vi "数据查询_仪器数据.vi"() -> ()   [LabVIEW 2016]
uses:
  <vilib>/Utility/miscctls.llb/LVPointTypeDef.ctl
  <vilib>/Utility/miscctls.llb/LVRowAndColumnUnsignedTypeDef.ctl
  <userlib>/_OpenG.lib/array/array.llb/Sort 2D Array (String)__ogtk.vi
panel:
  in  "序列号":string
  in  "关闭":bool
  in  "导出":bool
  out "分钟小时":string(combo)="实时数据"
  out "工作类型":string(combo)="全部数据"
  in  "工作模式":string(combo)="全部数据"
  in  "查询":bool
  in  "结束日期":string="2020/01/01"
  in  "起始日期":string="2010/01/01"
  in  "组合框":string(combo)
  out "数据表":string[][](table)
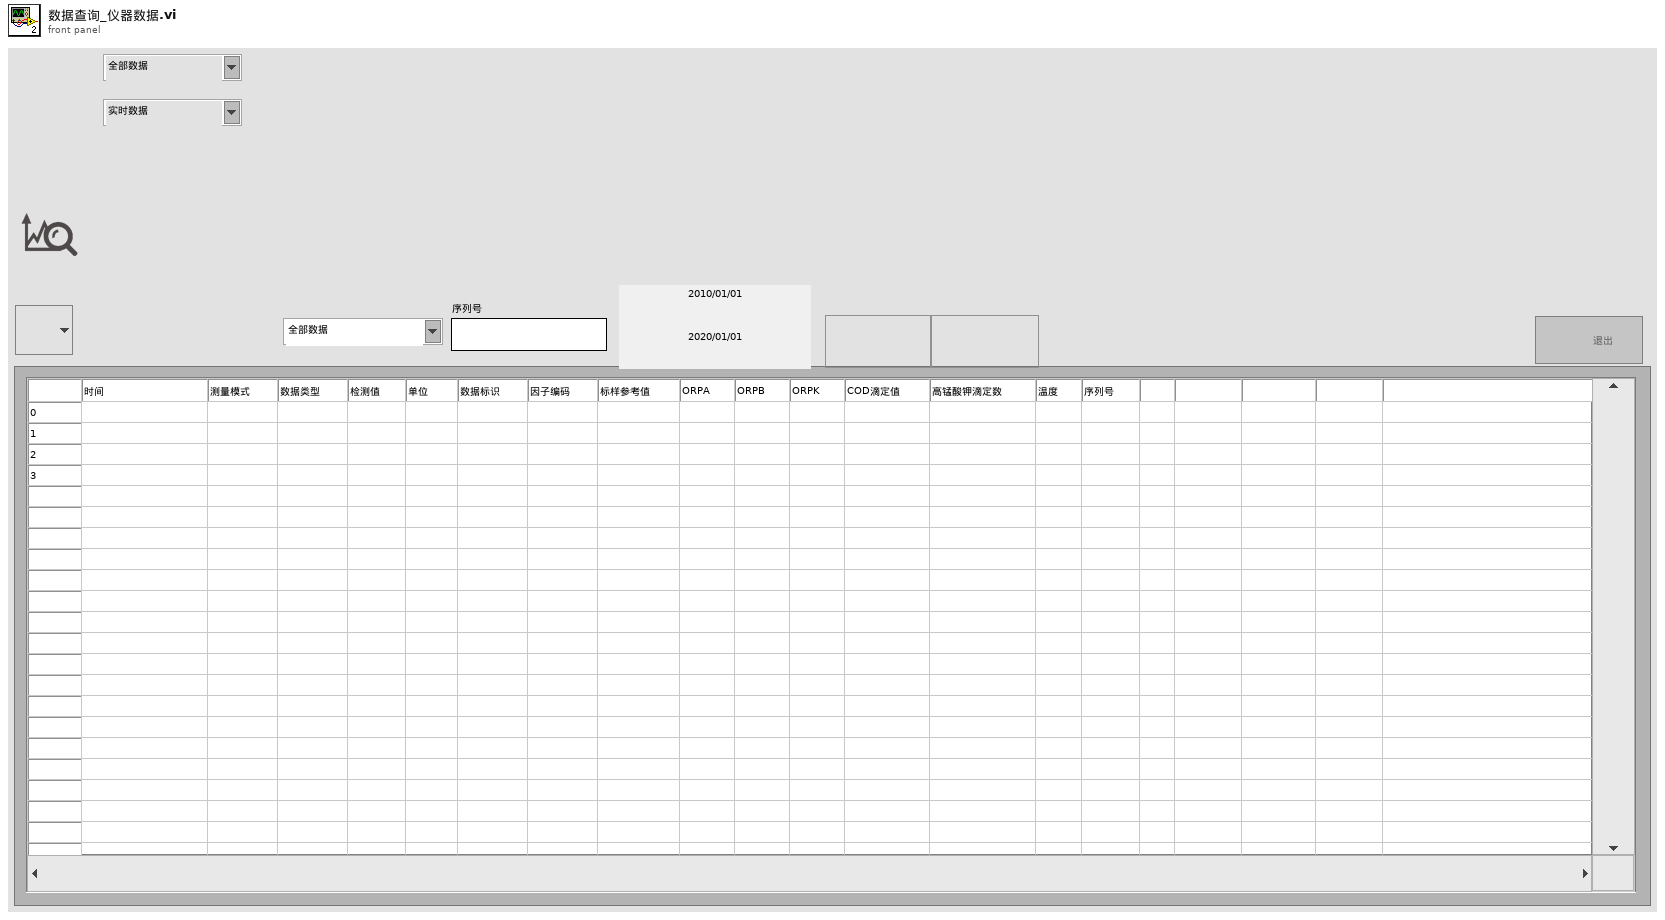
[diagram p1: front panel]
types:
  T1 = enum8{"Enabled", "Disabled", "Disabled and Grayed Out"}
  T2 = typedef "LVRowAndColumnUnsignedTypeDef.ctl" = cluster{"Row":u32, "Column":u32}
  T3 = typedef "LVPointTypeDef.ctl" = cluster{"Horizontal":i16, "Vertical":i16}
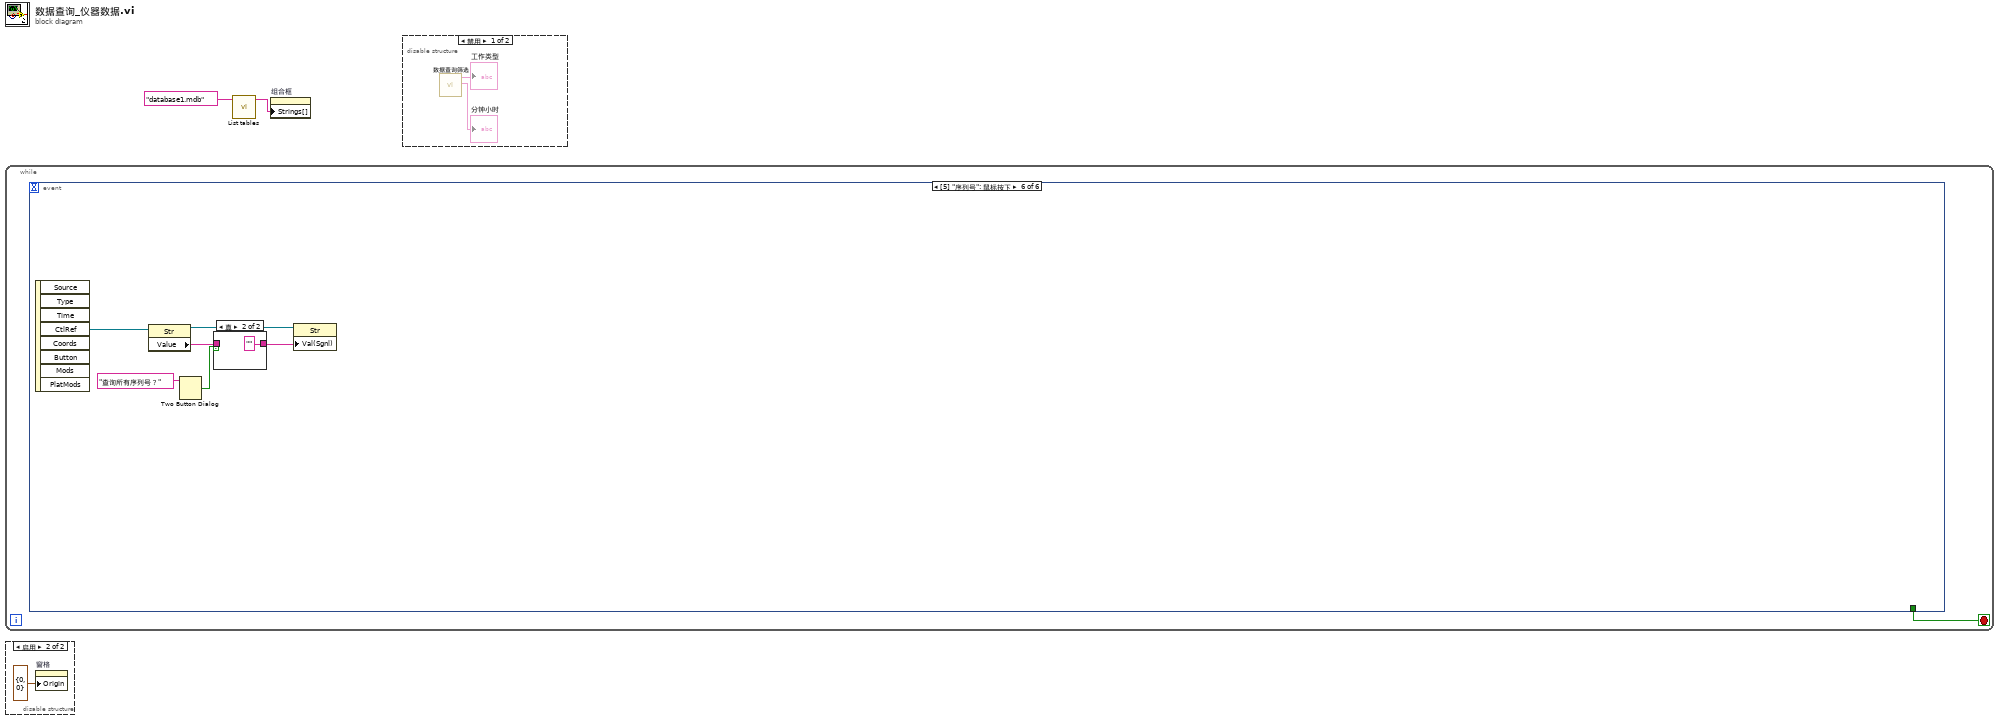
[diagram p0: block diagram]
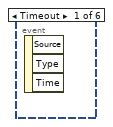
[diagram p3: hidden frame]
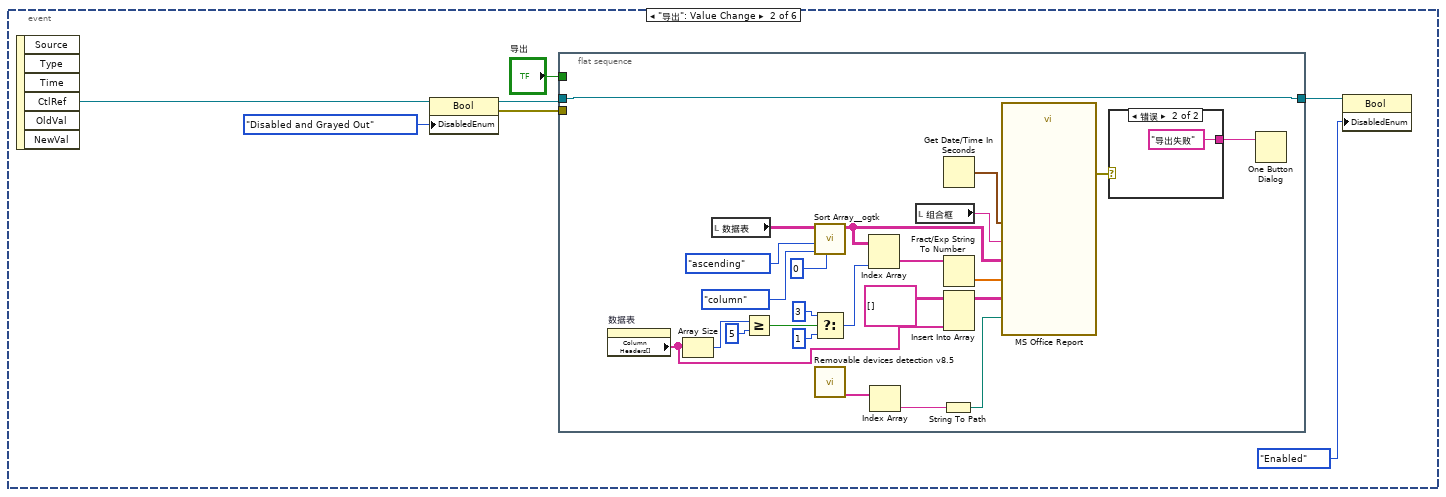
[diagram p4: hidden frame]
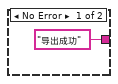
[diagram p5: hidden frame]
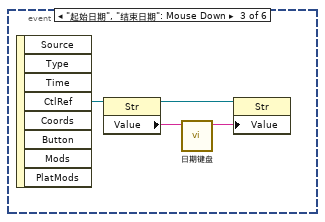
[diagram p6: hidden frame]
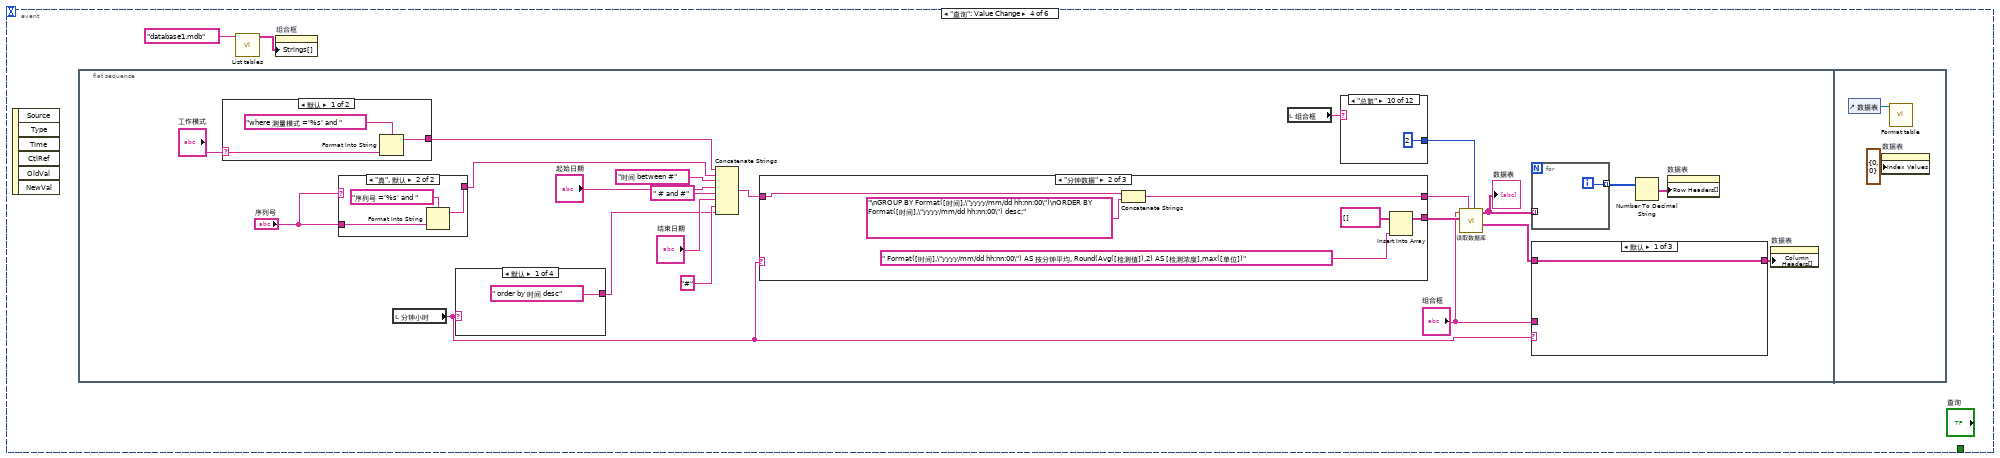
[diagram p7: hidden frame]
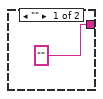
[diagram p8: hidden frame]
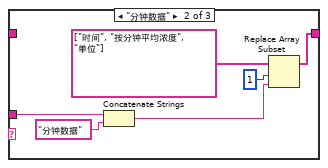
[diagram p9: hidden frame]
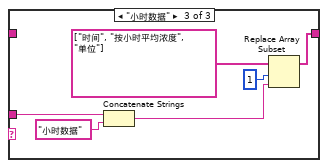
[diagram p10: hidden frame]
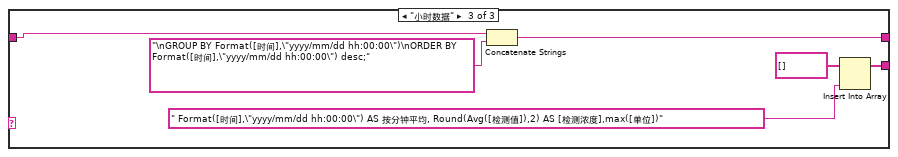
[diagram p15: hidden frame]
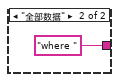
[diagram p16: hidden frame]
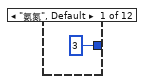
[diagram p17: hidden frame]
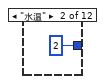
[diagram p18: hidden frame]
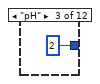
[diagram p19: hidden frame]
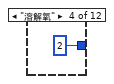
[diagram p20: hidden frame]
diagram:
  n1 = while {
    stop <- w3 stop-if-true
    n2 = event shown="[5] \"序列号\": 鼠标按下" {
      selector: _ -> [_ _ _ _ _ _]
      dyn-events: _ -> [_ _ _ _ _ _]
      timeout: _ -> [_ _ _ _ _ _]
      tunnel: [_ _ _ _ TRUE ("停止？(T)") _] -> w3
      event Timeout {
        n3 = event-data() -> ()  [unwired: 1 in, 3 out]
      }
      event "导出": Value Change {
        n4 = event-data() -> ("CtlRef"=w4:refnum<vi>)  [unwired: 1 in, 5 out]
        n5 = property class="Bool"(reference=w4, "DisabledEnum"=T1."Disabled and Grayed Out" ("禁用")) -> (reference out=w8:refnum<vi>, error out=w9:errorcluster)  [unwired: 1 in]
        n6 = flat-sequence {
          tunnel: w9 -> [_]
          tunnel: [w25] -> w7
          tunnel: w8 -> [w25]
          tunnel: "导出" -> [_]
          frame #0 {
            n7 = property on="数据表" class="Tbl (严格)"() -> ("Column Headers[]"=w12:string[])  [unwired: 2 in, 2 out]
            n8 = Array Size(array=w12) -> (size(s)=w19:i32)
            n9 = local read "数据表"() -> (w33:string[][])
            n10 = Greater Or Equal?(x=w19, y=5) -> (x >= y?=w17:bool)
            n11 = call-poly <userlib>:"Sort Array__ogtk.vi"("Column/Row to Sort By"=u32 0, "Sort By in"=enum16{"row", "column"}."column", "Order"=enum16{"ascending", "descending"}."ascending", "Array in"=w33) -> ("Sorted Array out"=w32:string[][])  [unwired: 4 in, 3 out]
            n12 = Select(t=3 ("禁用的索引 (列)"), s=w17, f=1) -> (s? t:f=w15:i32)
            n13 = call "Removable devices detection v8.5.vi"() -> ("Removable"=w22:string[])  [unwired: 4 out]
            n14 = Index Array(array=w32, index (col)=w15) -> (element=w28:string[])  [unwired: 1 in]
            n15 = Index Array(array=w22) -> (element=w21:string)  [unwired: 1 in]
            n16 = local read "组合框"() -> (w26:string)
            n17 = String To Path(string=w21) -> (path=w20:path)
            n18 = Get Date/Time In Seconds() -> (seconds since 1Jan1904=w34:timestamp)
            n19 = Fract/Exp String To Number(string=w28) -> (number=w27:dbl[])  [unwired: 3 in, 1 out]
            n20 = Insert Into Array(array=string[][] [], new element=w12) -> (w11:string[][])  [unwired: 2 in]
            n21 = call "MS Office Report"("Path to Save Report"=w20, "导出日期"=w34, "监测参数"=w26, "数据输入"=w32, "图表输入"=w27, "字段定义"=w11) -> ("error out"=w24:errorcluster)  [unwired: 20 in, 1 out]
            n22 = case shown="错误" w24 {
              tunnel: ["导出成功" ("消息") "导出失败" ("消息")] -> w23
              frame No Error {
              }
              frame Error {
              }
            }
            n23 = One Button Dialog(message=w23) -> ()  [unwired: 1 in, 1 out]
          }
        }
        n24 = property class="Bool"(reference=w7, "DisabledEnum"=T1."Enabled" ("禁用")) -> ()  [unwired: 1 in, 2 out]
      }
      event "起始日期", "结束日期": Mouse Down {
        n25 = event-data() -> ("CtlRef"=w40:refnum<vi>)  [unwired: 1 in, 7 out]
        n26 = property class="Str"(reference=w40) -> (reference out=w38:refnum<vi>, "Value"=w39:string)  [unwired: 1 in, 1 out]
        n27 = call "日期键盘.vi"("原值"=w39) -> ("x+y"=w37:string)  [unwired: 10 in]
        n28 = property class="Str"(reference=w38, "Value"=w37) -> ()  [unwired: 1 in, 2 out]
      }
      event "查询": Value Change {
        n29 = event-data() -> ()  [unwired: 1 in, 6 out]
        n30 = flat-sequence {
          frame #0 {
            n31 = case shown="默认" "工作模式" {
              selector: "工作模式" -> [w98 _]
              tunnel: [w96 "where " ("condition")] -> w44
              frame Default {
                n32 = Format Into String(format string="where 测量模式 ='%s' and " ("condition"), w98) -> (resulting string=w96:string)  [unwired: 2 in, 1 out]
              }
              frame "全部数据" {
              }
            }
            n33 = case shown="\"真\", 默认" "序列号" {
              tunnel: "序列号" -> [_ w67]
              tunnel: ["" ("condition") w66] -> w43
              frame "" {
              }
              frame "真", Default {
                n34 = Format Into String(format string="序列号 ='%s' and " ("condition"), w67) -> (resulting string=w66:string)  [unwired: 2 in, 1 out]
              }
            }
            n35 = local read "分钟小时"() -> (w51:string)
            n36 = case shown="默认" w51 {
              tunnel: [" order by 时间 desc" ("字符串") _ _ _] -> w55
              frame Default {
              }
              frame "分钟数据" {
              }
              frame "小时数据" {
              }
              frame "真" {
              }
            }
            n37 = Concatenate Strings(w44, w43, "时间 between #" ("condition"), "起始日期", " # and #" ("condition"), "结束日期", "#" ("condition"), w55) -> (w54:string)
            n38 = case shown="\"分钟数据\"" w51 {
              tunnel: [_ w88 w90] -> w52
              tunnel: w54 -> [w83 w86 w92]
              tunnel: [w83 w85 w91] -> w53
              frame Default {
              }
              frame "分钟数据" {
                n39 = Concatenate Strings(w86, "\nGROUP BY Format([时间],\"yyyy/mm/dd hh:nn:00\")\nORDER BY Format([时间],\"yyyy/mm/dd hh:nn:00\") desc;" ("字符串")) -> (w85:string)
                n40 = Insert Into Array(array=string[] [] ("显示项"), new element=" Format([时间],\"yyyy/mm/dd hh:nn:00\") AS 按分钟平均, Round(Avg([检测值]),2) AS [检测浓度],max([单位])" ("新元素/子数组")) -> (w88:string[])  [unwired: 1 in]
              }
              frame "小时数据" {
                n41 = Concatenate Strings(w92, "\nGROUP BY Format([时间],\"yyyy/mm/dd hh:00:00\")\nORDER BY Format([时间],\"yyyy/mm/dd hh:00:00\") desc;" ("字符串")) -> (w91:string)
                n42 = Insert Into Array(array=string[] [] ("显示项"), new element=" Format([时间],\"yyyy/mm/dd hh:00:00\") AS 按分钟平均, Round(Avg([检测值]),2) AS [检测浓度],max([单位])" ("新元素/子数组")) -> (w90:string[])  [unwired: 1 in]
              }
            }
            n43 = local read "组合框"() -> (w57:string)
            n44 = case shown="\"总氮\"" w57 {
              tunnel: [i16 3 ("精度(6)") i16 2 ("精度(6)") i16 2 ("精度(6)") i16 2 ("精度(6)") i16 2 ("精度(6)") i16 2 ("精度(6)") i16 2 ("精度(6)") i16 2 ("精度(6)") i16 3 ("精度(6)") i16 2 ("精度(6)") i16 2 ("精度(6)") i16 2 ("精度(6)")] -> w56
              frame "氨氮", Default {
              }
              frame "水温" {
              }
              frame "pH" {
              }
              frame "溶解氧" {
              }
              frame "电导率" {
              }
              frame "浊度" {
              }
              frame "藻密度" {
              }
              frame "叶绿素a" {
              }
              frame "总磷" {
              }
              frame "总氮" {
              }
              frame "CodCr" {
              }
              frame "CodMn" {
              }
            }
            n45 = call "读取数据库.vi"("精度(6)"=w56, "condition"=w53, "显示项"=w52, "组合框"="组合框") -> ("columns"=w50:string[], "表格"=w60:string[][])  [unwired: 4 in, 2 out]
            "数据表" <- w60
            n46 = for {
              tunnel: w60 -> [_] mode=indexing
              tunnel: [w112] -> w59 mode=indexing
              i -> [w112]
            }
            n47 = case shown="默认" w51 {
              tunnel: w50 -> [w69 _ _]
              tunnel: [w69 w73 w77] -> w49
              tunnel: "组合框" -> [_ w72 w78]
              frame Default {
              }
              frame "分钟数据" {
                n48 = Concatenate Strings(w72, "分钟数据" ("字符串")) -> (w70:string)
                n49 = Replace Array Subset(array=string[] ["时间", "按分钟平均浓度", "单位"] ("columns"), new element=w70, index=1 ("索引")) -> (w73:string[])
              }
              frame "小时数据" {
                n50 = Concatenate Strings(w78, "小时数据" ("字符串")) -> (w79:string)
                n51 = Replace Array Subset(array=string[] ["时间", "按小时平均浓度", "单位"] ("columns"), new element=w79, index=1 ("索引")) -> (w77:string[])
              }
            }
            n52 = Number To Decimal String(number=w59) -> (decimal integer string=w58:string[])  [unwired: 1 in]
            n53 = property on="数据表" class="Tbl (严格)"("Row Headers[]"=w58) -> ()  [unwired: 2 in, 2 out]
            n54 = property on="数据表" class="Tbl (严格)"("Column Headers[]"=w49) -> ()  [unwired: 2 in, 2 out]
          }
          frame #1 {
            n55 = control-ref of="数据表"() -> (w113:refnum<vi>)
            n56 = property on="数据表" class="Tbl (严格)"("Index Values"=T2 {"Row"=0, "Column"=0} ("索引值")) -> ()  [unwired: 2 in, 2 out]
            n57 = call "Format table.vi"("Table输入"=w113) -> ()  [unwired: 11 in]
          }
        }
        n58 = call "List tables.vi"("database"="database1.mdb") -> ("tables"=w42:string[])  [unwired: 9 in, 1 out]
        n59 = property on="组合框" class="CmbBox"("Strings[]"=w42) -> ()  [unwired: 2 in, 2 out]
      }
      event Panel Close; "关闭": Value Change {
        n60 = event-data() -> ()  [unwired: 1 in, 3 out]
      }
      event "序列号": Mouse Down {
        n61 = event-data() -> ("CtlRef"=w121:refnum<vi>)  [unwired: 1 in, 7 out]
        n62 = property class="Str"(reference=w121) -> (reference out=w119:refnum<vi>, "Value"=w120:string)  [unwired: 1 in, 1 out]
        n63 = Two Button Dialog(message="查询所有序列号？" ("消息")) -> (T button?=w116:bool)  [unwired: 2 in]
        n64 = case shown="真" w116 {
          tunnel: w120 -> [w123 _]
          tunnel: [w122 "" ("x+y")] -> w118
          frame False {
            n65 = call "字符键盘.vi"("原值"=w123) -> ("x+y"=w122:string)  [unwired: 10 in]
          }
          frame True {
          }
        }
        n66 = property class="Str"(reference=w119, "Val(Sgnl)"=w118) -> ()  [unwired: 1 in, 2 out]
      }
    }
  }
  n67 = disable-structure shown="启用" {
    frame Disabled {
    }
    frame Enabled {
      n68 = property on="窗格" class="Pane"("Origin"=T3 {"Horizontal"=0, "Vertical"=0} ("原点")) -> ()  [unwired: 2 in, 2 out]
    }
  }
  n69 = call "List tables.vi"("database"="database1.mdb") -> ("tables"=w1:string[])  [unwired: 9 in, 1 out]
  n70 = property on="组合框" class="CmbBox"("Strings[]"=w1) -> ()  [unwired: 2 in, 2 out]
  n71 = disable-structure shown="禁用" {
    frame Disabled {
      n72 = call "数据查询筛选.vi"() -> ("分钟小时"=→"分钟小时":string, "工作类型"=→"工作类型":string)  [unwired: 10 in]
    }
    frame Enabled {
    }
  }
